vi "York DIHB - Legacy Software.vi"() -> ()   [LabVIEW 2020]
panel:
  in  "Timeout\nPeriod (s)":dbl=45.0
  out "Calculated\nVelocity":dbl
  out "Counter\n Value":dbl
  in  "Number of \nSamples":dbl=100000.0
  in  "Sample\n Rate":dbl=2000000.0
  out "Waveform Graph":dynamicdata(graph)
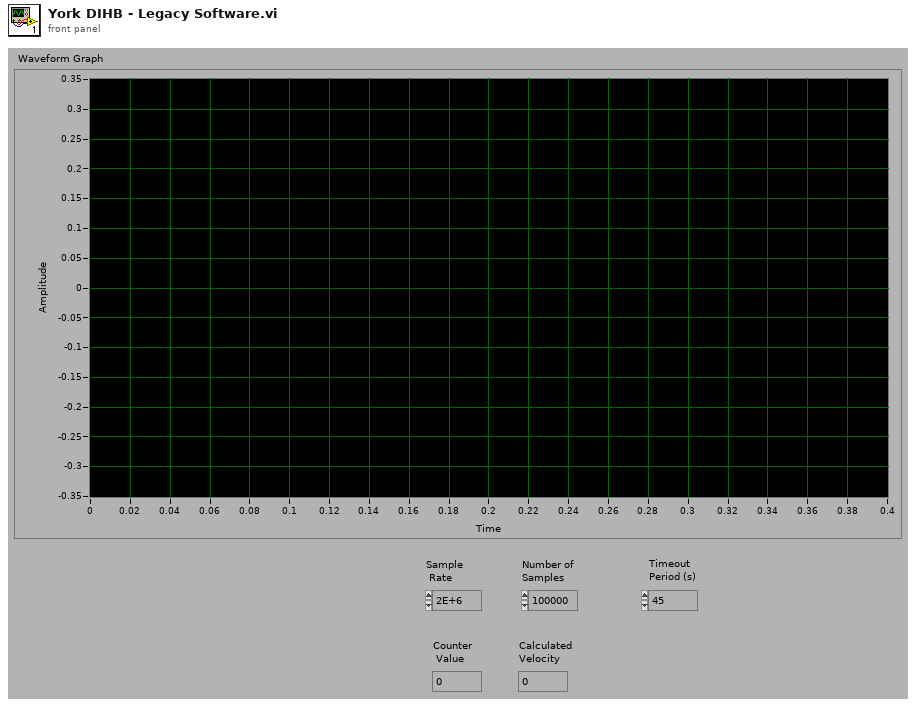
[diagram p1: front panel]
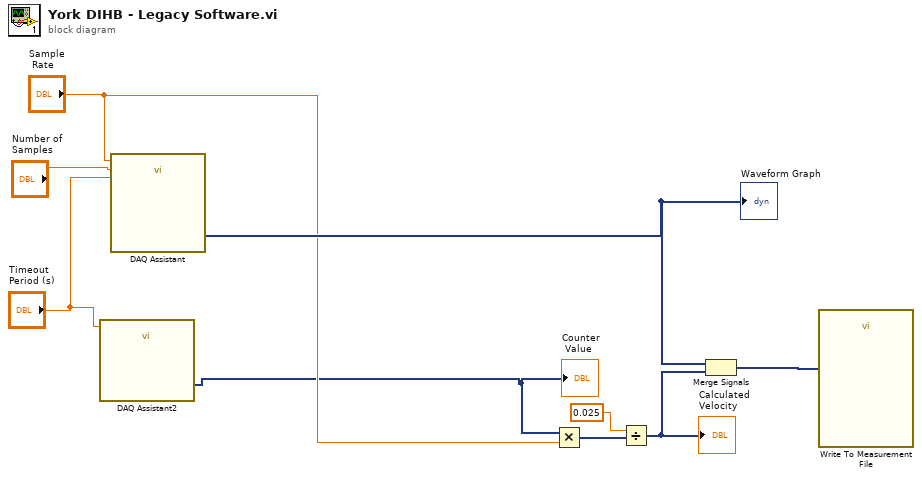
[diagram p0: block diagram]
diagram:
  n1 = call "DAQ Assistant2"("timeout (s)"="Timeout\nPeriod (s)") -> ("data"=w2:dynamicdata)  [unwired: 16 in, 2 out]
  "Counter\n Value" <- w2
  n2 = call "DAQ Assistant"("rate"="Sample\n Rate", "number of samples"="Number of \nSamples", "timeout (s)"="Timeout\nPeriod (s)") -> ("data"=w5:dynamicdata)  [unwired: 14 in, 2 out]
  "Waveform Graph" <- w5
  n3 = Multiply(x=w2, y="Sample\n Rate") -> (x*y=w9:dynamicdata)
  n4 = Divide(x=0.025, y=w9) -> (x/y=w6:dynamicdata)
  "Calculated\nVelocity" <- w6
  n5 = Merge Signals(w5, w6) -> (w7:dynamicdata)
  n6 = call "Write To Measurement File"("Signals"=w7) -> ()  [unwired: 16 in, 3 out]
